vi "Write settings.vi"(8 "error in (no error)":errorcluster, 10 "settings name in":string, 11 "Trace in":refnum<class "Trace.lvclass">) -> (0 "error out":errorcluster, 2 "settings name out":string, 3 "Trace out":refnum<class "Trace.lvclass">)   [LabVIEW 2012, in "Trace.lvclass"]
doc: "Writes the settings cluster into the settings file. Settings file is XML-based. It's name is <component ID>.xml"
uses:
  Trace.lvclass
  <vilib>/Distrio/Murmex/Murmex/Murmex.lvclass
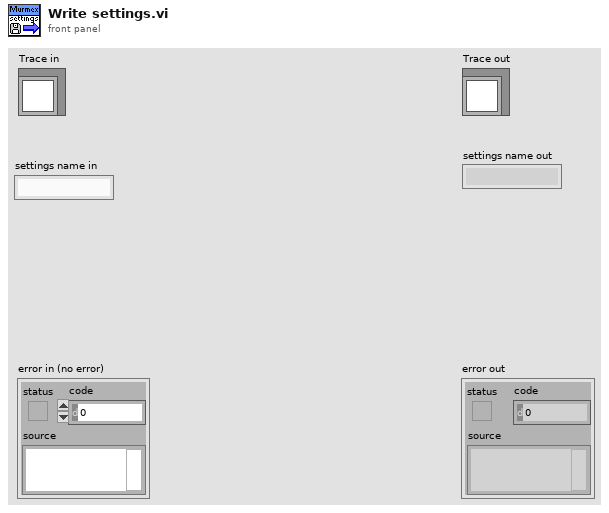
[diagram p1: front panel]
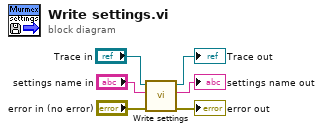
[diagram p0: block diagram]
diagram:
  n1 = call-parent "Write settings.vi"("error in (no error)"="error in (no error)", "settings name in"="settings name in", "Murmex in"="Trace in") -> ("error out"=→"error out":errorcluster, "settings name out"=→"settings name out":string, "Murmex out"=→"Trace out":refnum<class "Trace.lvclass">)  [unwired: 6 in]
